vi "setREF_RollOff.vi"(8 "error in (no error)":errorcluster, 9 "Roll-Off":i32=1 min=1, 10 "REF Channel":i32=1 min=1 max=16, 11 "Instrument.LockinAPI in":refnum<class "Instrument.LockinAPI.lvclass">) -> (0 "error out":errorcluster, 3 "Instrument.LockinAPI out":refnum<class "Instrument.LockinAPI.lvclass">)   [LabVIEW 2019, in "Instrument.LockinAPI.lvclass"]
doc: "API to configure a REF frequency.\n\nSpecify which channel you want to change and the value you want to set.\n\nIf address=\"\", this API reads from localhost\nIf address is remote lockin, you need to add this computer to allowed whitelist on the lockin computer you are trying to access."
uses:
  Instrument.LockinAPI.lvclass
  Typedefs/API/LockinAPI.Commands--Enum.ctl
  97eaa401-7be6-42d3-beed-c4ab4e0956cc.vi
  Typedefs/API/LockinAPI.setREF_RollOff--cluster.ctl
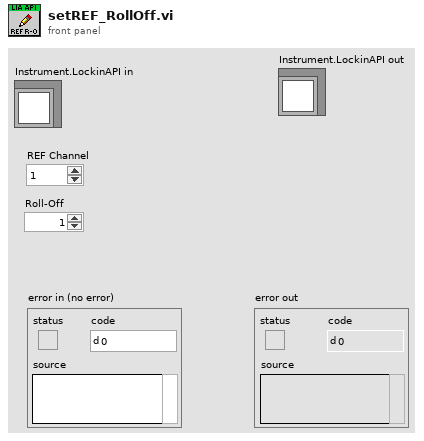
[diagram p1: front panel]
types:
  T1 = typedef "Instrument.LockinAPI.lvclass/LockinAPI.setREF_RollOff--cluster.ctl" = cluster{"REF Channel":i32, "Roll-Off":i32}
  T2 = typedef "Instrument.LockinAPI.lvclass/LockinAPI.Commands--Enum.ctl" = enum16{"setAI", "setAO", "setAO_Amplitude", "setAO_DC", "setAO_Frequency", "setAO_Phase", "setAO_Function", "setAO_I+", "setREF", "setREF_Frequency", "setREF_Phase", "setREF_TC", "setREF_Roll-Off", "setDAQ", "setSampling", "setOffset", "setState", "getState", "getAO", "getAI", "getResults", "getSampling", "getAOconfig", "getREFconfig", "setInputGain", "setOutputGain", "getInputGain", "getOutputGain", "setSamplingMode", "getSamplingMode", "setSweep", "setSweepTime", "setSweepTable", "getStatus", "getSweepResults", "getSweepWaveforms", "startSweep", "stopSweep", "setAUX", "getAUX"}
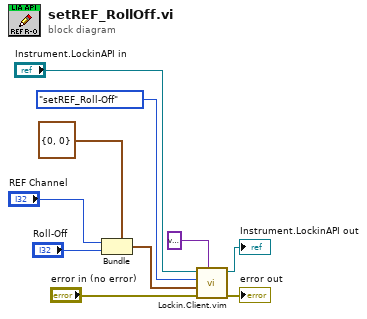
[diagram p0: block diagram]
diagram:
  n1 = Bundle(cluster=T1 {"REF Channel"=0, "Roll-Off"=0} ("setREF_phi"), "REF Channel"="REF Channel", "Roll-Off"="Roll-Off") -> (w4:T1)
  n2 = call "Lockin.Client.vim"("Data Out type"=variant, "error in (no error)"="error in (no error)", "Data"=w4, "Command"=LockinAPI.Commands--Enum."setREF_Roll-Off", "Instrument.LockinAPI in"="Instrument.LockinAPI in") -> ("error out"=→"error out":errorcluster, "Instrument.LockinAPI out"=→"Instrument.LockinAPI out":refnum<class "Instrument.LockinAPI.lvclass">)  [unwired: 4 in, 1 out]
